vi "CFU_5p2_jones6sv.vi"() -> ()   [LabVIEW 2016]
uses:
  <vilib>/express/express arith-compare/Formula/XNode/ExpressFormulaBlockNode.xnode
  <vilib>/express/express shared/transition.llb/Dynamic To Waveform Array.vi
  <vilib>/express/express arith-compare/Formula/Block/exnFormulaBlock how many pts in the wave.vi
  <vilib>/express/express shared/ex_Modify Signal Name.vi
  <vilib>/express/express shared/transition.llb/Waveform Array To Dynamic.vi
panel:
  out "Total R":dbl
  in  "R2":dbl
  in  "R1":dbl
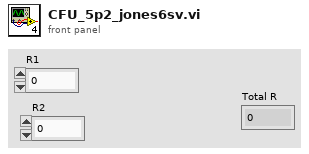
[diagram p1: front panel]
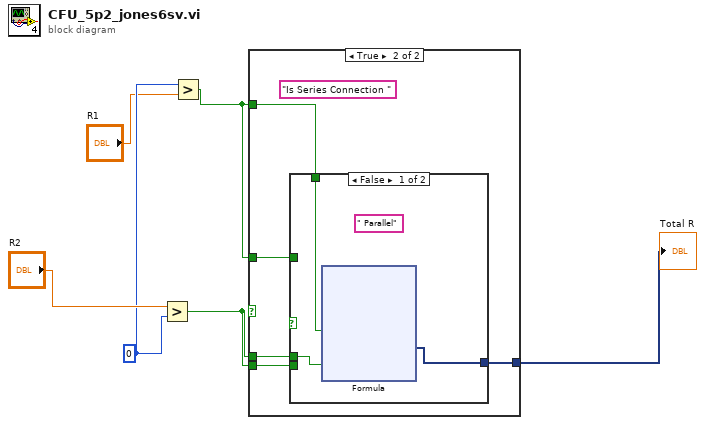
[diagram p0: block diagram]
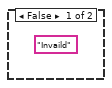
[diagram p2: hidden frame]
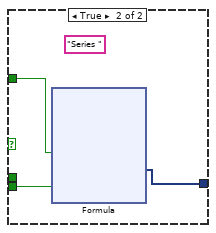
[diagram p3: hidden frame]
diagram:
  w5 = 0
  n1 = Greater?(x="R2", y=w5) -> (0:w1:bool)
  n2 = Greater?(x=w5, y="R1") -> (0:w2:bool)
  n3 = case shown="True" {
    selector: _ -> [_ _]
    tunnel: [_ w11] -> w3
    tunnel: w2 -> [_ w10]
    tunnel: w1 -> [_ w9]
    tunnel: w2 -> [_ w8]
    tunnel: w1 -> [_ w7]
    frame False {
      (unwired) "Invaild"
    }
    frame True {
      (unwired) "Is Series Connection "
      n4 = case shown="False" {
        selector: _ -> [_ _]
        tunnel: [w12 w156] -> w11
        tunnel: w10 -> [_ w155]
        tunnel: w9 -> [_ w154]
        tunnel: w8 -> [w14 _]
        tunnel: w7 -> [w13 _]
        frame False {
          (unwired) " Parallel"
          n5 = xnode "Formula"("R1"=w14, "R2"=w13) -> ("Result"=w12:dynamicdata)  [unwired: 1 in, 1 out]
        }
        frame True {
          (unwired) "Series "
          n6 = xnode "Formula"("R1"=w155, "R2"=w154) -> ("Result"=w156:dynamicdata)  [unwired: 1 in, 1 out]
        }
      }
    }
  }
  "Total R" <- w3
